vi "Stop Logging.vi"() -> (0 "error out":errorcluster, 1 "completed log files":string[](array[string]))   [LabVIEW 2015]
uses:
  <vilib>/NI Veristand/Execution/DataLogging/NI_VS Data Logging API.lvlib
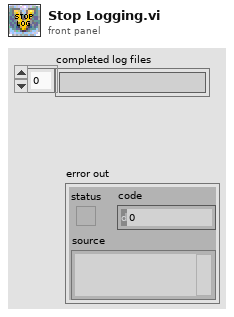
[diagram p1: front panel]
types:
  T1 = typedef "NI_VS Data Logging API.lvlib/IDataLogging Ref.ctl" = refnum<k24>
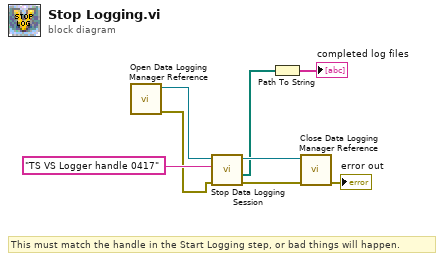
[diagram p0: block diagram]
diagram:
  # "This must match the handle in the Start Logging step, or bad things will happen."
  n1 = call <vilib>:"Open Data Logging Manager Reference.vi"() -> ("error out"=w2:errorcluster, "Data Logging Manager Ref out"=w3:T1)  [unwired: 10 in]
  n2 = call <vilib>:"Stop Data Logging Session.vi"("error in (no error)"=w2, "Session Name in"="TS VS Logger handle 0417" ("Logging Session Name in"), "Data Logging Manager Ref in"=w3) -> ("error out"=w6:errorcluster, "Log File Paths"=w4:path[], "Data Logging Manager Ref out"=w8:T1)  [unwired: 5 in, 1 out]
  n3 = Path To String(path=w4) -> (string=→"completed log files":string[])
  n4 = call <vilib>:"Close Data Logging Manager Reference.vi"("error in (no error)"=w6, "Data Logging Manager Ref in"=w8) -> ("error out"=→"error out":errorcluster)  [unwired: 9 in]
